vi "5492_LiftButtons.vi"() -> ()   [LabVIEW 2017]
panel:
  in  "Manual":dbl
  in  "Collect Set":dbl
  in  "Low set":dbl
  in  "High Set":dbl
  in  "Collect":bool
  in  "Lo":bool
  in  "Hi":bool
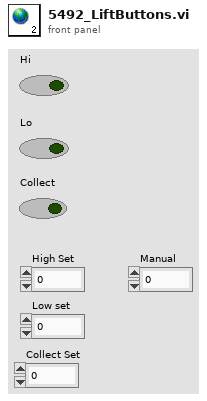
[diagram p1: front panel]
diagram:
